vi "Generate Topic Rule JSON.vi"(11 "Topic Rule":T1) -> (3 "Topic Rule JSON":string)   [LabVIEW 2015, in "NI_AWS_IoT.lvlib"]
uses:
  NI_AWS_IoT.lvlib
  Topic Rule.ctl
  CloudWatch Alarm.ctl
  CloudWatch Metric.ctl
  DynamoDB.ctl
  DynamoDBv2.ctl
  Elasticsearch.ctl
  Firehose.ctl
  Kinesis.ctl
  Lambda.ctl
  Republish.ctl
  S3.ctl
  SNS.ctl
  SQS.ctl
  JSON Parsing/NI_JSON Parsing.lvlib
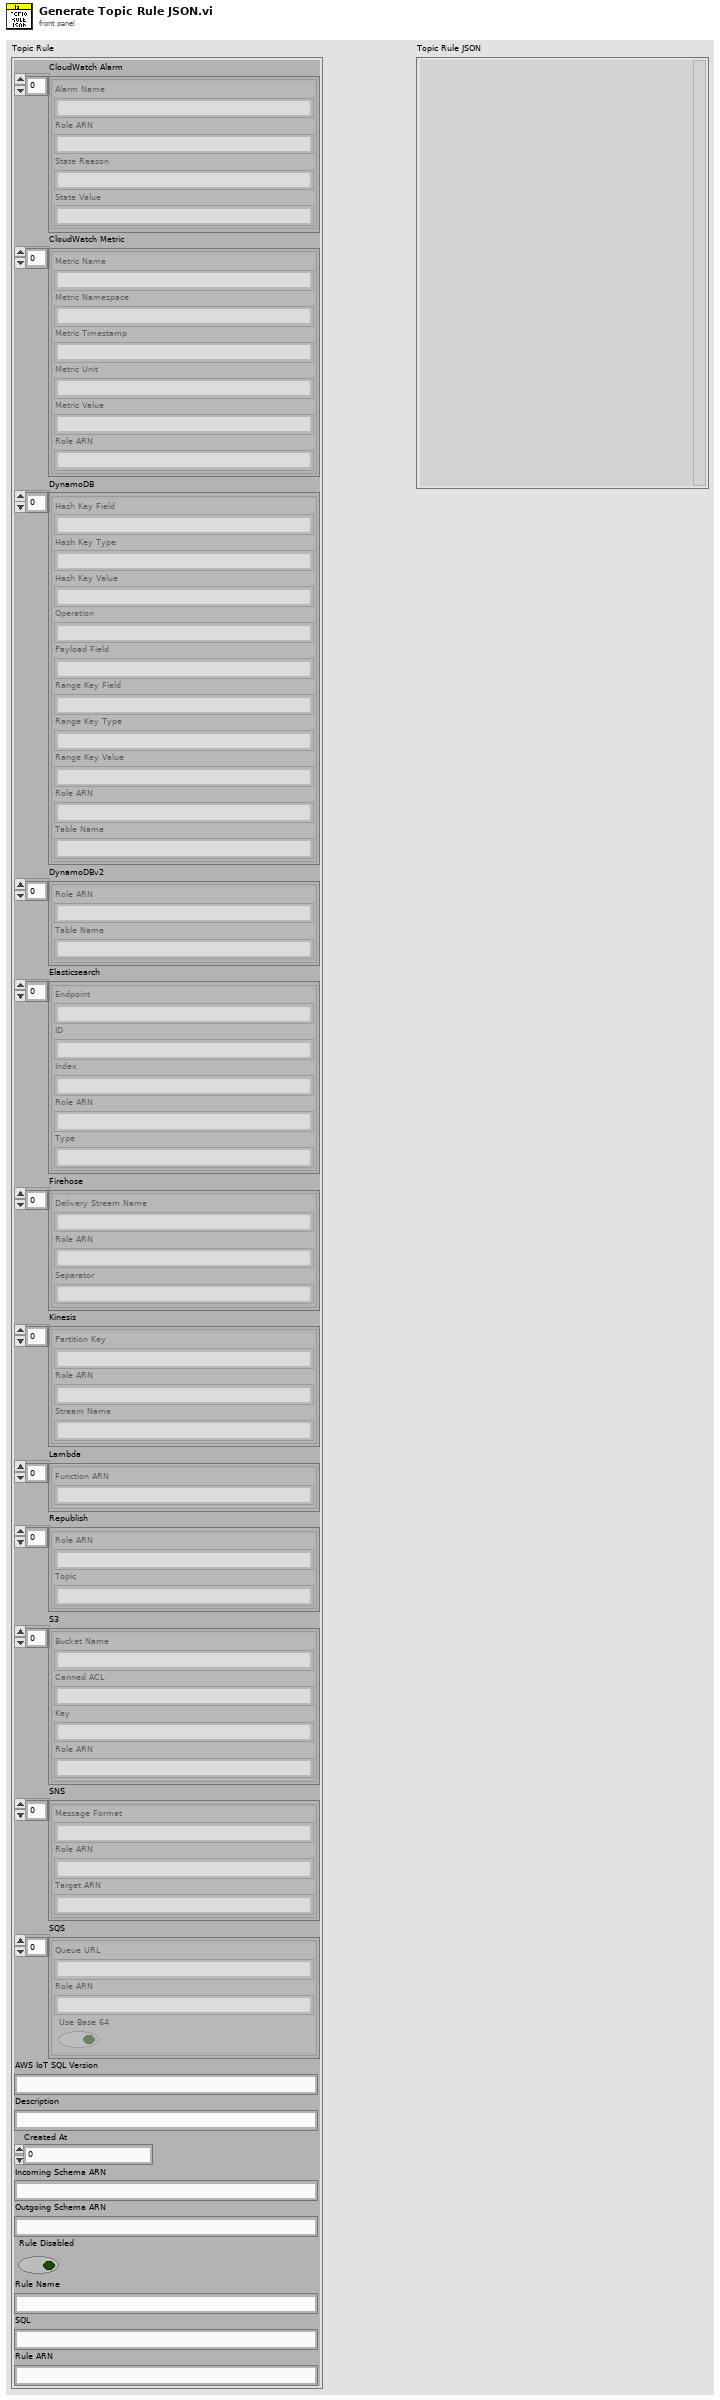
[diagram p1: front panel]
types:
  T1 = typedef "NI_AWS_IoT.lvlib/Topic Rule.ctl" = cluster{"CloudWatch Alarm":T2[], "CloudWatch Metric":T3[], "DynamoDB":T4[], "DynamoDBv2":T5[], "Elasticsearch":T6[], "Firehose":T7[], "Kinesis":T8[], "Lambda":T9[], "Republish":T10[], "S3":T11[], "SNS":T12[], "SQS":T13[], "AWS IoT SQL Version":string, "Description":string, "Created At":u64, "Incoming Schema ARN":string, "Outgoing Schema ARN":string, "Rule Disabled":bool, "Rule Name":string, "SQL":string, "Rule ARN":string}
  T2 = typedef "NI_AWS_IoT.lvlib/CloudWatch Alarm.ctl" = cluster{"Alarm Name":string, "Role ARN":string, "State Reason":string, "State Value":string}
  T3 = typedef "NI_AWS_IoT.lvlib/CloudWatch Metric.ctl" = cluster{"Metric Name":string, "Metric Namespace":string, "Metric Timestamp":string, "Metric Unit":string, "Metric Value":string, "Role ARN":string}
  T4 = typedef "NI_AWS_IoT.lvlib/DynamoDB.ctl" = cluster{"Hash Key Field":string, "Hash Key Type":string, "Hash Key Value":string, "Operation":string, "Payload Field":string, "Range Key Field":string, "Range Key Type":string, "Range Key Value":string, "Role ARN":string, "Table Name":string}
  T5 = typedef "NI_AWS_IoT.lvlib/DynamoDBv2.ctl" = cluster{"Role ARN":string, "Table Name":string}
  T6 = typedef "NI_AWS_IoT.lvlib/Elasticsearch.ctl" = cluster{"Endpoint":string, "ID":string, "Index":string, "Role ARN":string, "Type":string}
  T7 = typedef "NI_AWS_IoT.lvlib/Firehose.ctl" = cluster{"Delivery Stream Name":string, "Role ARN":string, "Separator":string}
  T8 = typedef "NI_AWS_IoT.lvlib/Kinesis.ctl" = cluster{"Partition Key":string, "Role ARN":string, "Stream Name":string}
  T9 = typedef "NI_AWS_IoT.lvlib/Lambda.ctl" = cluster{"Function ARN":string}
  T10 = typedef "NI_AWS_IoT.lvlib/Republish.ctl" = cluster{"Role ARN":string, "Topic":string}
  T11 = typedef "NI_AWS_IoT.lvlib/S3.ctl" = cluster{"Bucket Name":string, "Canned ACL":string, "Key":string, "Role ARN":string}
  T12 = typedef "NI_AWS_IoT.lvlib/SNS.ctl" = cluster{"Message Format":string, "Role ARN":string, "Target ARN":string}
  T13 = typedef "NI_AWS_IoT.lvlib/SQS.ctl" = cluster{"Queue URL":string, "Role ARN":string, "Use Base 64":bool}
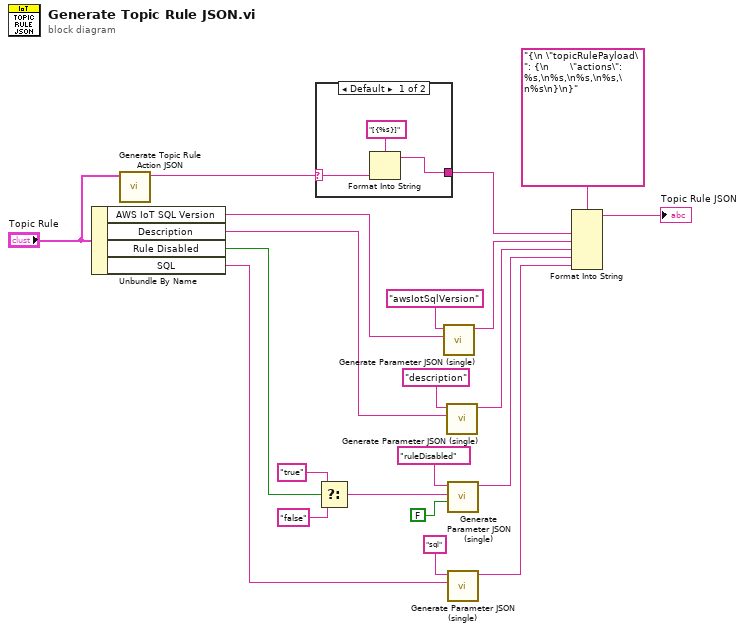
[diagram p0: block diagram]
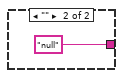
[diagram p2: hidden frame]
diagram:
  n1 = Unbundle By Name("Topic Rule") -> ("AWS IoT SQL Version"=w13:string, "Description"=w10:string, "Rule Disabled"=w8:bool, "SQL"=w3:string)
  n2 = call "Generate Topic Rule Action JSON.vi"("Topic Rule"="Topic Rule") -> ("Action JSON"=w16:string)  [unwired: 10 in]
  n3 = case shown="Default" w16 {
    selector: w16 -> [w24 _]
    tunnel: [w22 "null"] -> w15
    frame Default {
      n4 = Format Into String(format string="[{%s}]", w24) -> (resulting string=w22:string)  [unwired: 2 in, 1 out]
    }
    frame "" {
    }
  }
  n5 = Select(t="true", s=w8, f="false") -> (s? t:f=w6:string)
  n6 = call "Generate Parameter JSON (single).vi"("Parameter Value"=w13, "Parameter Name"="awsIotSqlVersion") -> ("Parameter JSON"=w12:string)  [unwired: 9 in]
  n7 = call "Generate Parameter JSON (single).vi"("Parameter Value"=w10, "Parameter Name"="description") -> ("Parameter JSON"=w9:string)  [unwired: 9 in]
  n8 = call "Generate Parameter JSON (single).vi"("Value in Quotes"=FALSE, "Parameter Value"=w6, "Parameter Name"="ruleDisabled") -> ("Parameter JSON"=w5:string)  [unwired: 8 in]
  n9 = call "Generate Parameter JSON (single).vi"("Parameter Value"=w3, "Parameter Name"="sql") -> ("Parameter JSON"=w2:string)  [unwired: 9 in]
  n10 = Format Into String(format string="{\n \"topicRulePayload\": {\n       \"actions\": %s,\n%s,\n%s,\n%s,\n%s\n}\n}", w15, w12, w9, w5, w2) -> (resulting string=→"Topic Rule JSON":string)  [unwired: 2 in, 1 out]
